vi "DICOMFormatToName.vi"(11 "DICOM Format Name":string) -> (3 "Name":string)   [LabVIEW 2013, in "main.lvlib"]
uses:
  main.lvlib
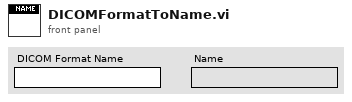
[diagram p1: front panel]
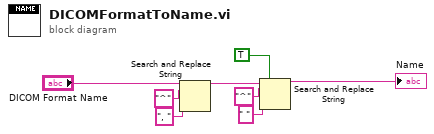
[diagram p0: block diagram]
diagram:
  n1 = Search and Replace String(input string="DICOM Format Name", search string="^" ("regular expression"), replace string=", " ("replace string (\"\")")) -> (result string=w6:string)  [unwired: 5 in, 3 out]
  n2 = Search and Replace String(replace all?=TRUE ("replace all? (F)"), input string=w6, search string="^" ("regular expression"), replace string=" " ("replace string (\"\")")) -> (result string=→"Name":string)  [unwired: 4 in, 3 out]
